vi "Parameter aktivieren.vi"(11 "Ref Anzeige":refnum<vi>[](array[refnum])) -> ()   [LabVIEW 2020, in "Anlagengrenzwerte.lvlib"]
uses:
  Anlagengrenzwerte.lvlib
  Passwortverwaltung/FGV Passwort Aktion.ctl
  Passwortverwaltung/Passwort.lvlib
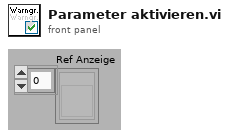
[diagram p1: front panel]
types:
  T1 = typedef "Passwort.lvlib/FGV Passwort Aktion.ctl" = enum16{"prüfen", "setzen", "Initialisieren", "PW speichern", "lesen", "PW Änderung"}
  T2 = cluster{cluster{"Soll aktiv":bool, "Warn Min aktiv":bool, "Warn Max aktiv":bool, "Abschalt Min aktiv":bool, "Abschalt Max aktiv":bool, "Regelung aktiv":bool}, cluster{"Soll aktiv":bool, "Warn Min aktiv":bool, "Warn Max aktiv":bool, "Abschalt Min aktiv":bool, "Abschalt Max aktiv":bool, "Regelung aktiv":bool}, cluster{"Soll aktiv":bool, "Warn Min aktiv":bool, "Warn Max aktiv":bool, "Abschalt Min aktiv":bool, "Abschalt Max aktiv":bool, "Regelung aktiv":bool}, cluster{"Soll aktiv":bool, "Warn Min aktiv":bool, "Warn Max aktiv":bool, "Abschalt Min aktiv":bool, "Abschalt Max aktiv":bool, "Regelung aktiv":bool}, cluster{"Soll aktiv":bool, "Warn Min aktiv":bool, "Warn Max aktiv":bool, "Abschalt Min aktiv":bool, "Abschalt Max aktiv":bool, "Regelung aktiv":bool}, cluster{"Soll aktiv":bool, "Warn Min aktiv":bool, "Warn Max aktiv":bool, "Abschalt Min aktiv":bool, "Abschalt Max aktiv":bool, "Regelung aktiv":bool}, cluster{"Soll aktiv":bool, "Warn Min aktiv":bool, "Warn Max aktiv":bool, "Abschalt Min aktiv":bool, "Abschalt Max aktiv":bool, "Regelung aktiv":bool}, cluster{"Soll aktiv":bool, "Warn Min aktiv":bool, "Warn Max aktiv":bool, "Abschalt Min aktiv":bool, "Abschalt Max aktiv":bool, "Regelung aktiv":bool}, cluster{"Soll aktiv":bool, "Warn Min aktiv":bool, "Warn Max aktiv":bool, "Abschalt Min aktiv":bool, "Abschalt Max aktiv":bool, "Regelung aktiv":bool}, cluster{"Soll aktiv":bool, "Warn Min aktiv":bool, "Warn Max aktiv":bool, "Abschalt Min aktiv":bool, "Abschalt Max aktiv":bool, "Regelung aktiv":bool}, cluster{"Soll aktiv":bool, "Warn Min aktiv":bool, "Warn Max aktiv":bool, "Abschalt Min aktiv":bool, "Abschalt Max aktiv":bool, "Regelung aktiv":bool}, cluster{"Soll aktiv":bool, "Warn Min aktiv":bool, "Warn Max aktiv":bool, "Abschalt Min aktiv":bool, "Abschalt Max aktiv":bool, "Regelung aktiv":bool}, cluster{"Soll aktiv":bool, "Warn Min aktiv":bool, "Warn Max aktiv":bool, "Abschalt Min aktiv":bool, "Abschalt Max aktiv":bool, "Regelung aktiv":bool}, cluster{"Soll aktiv":bool, "Warn Min aktiv":bool, "Warn Max aktiv":bool, "Abschalt Min aktiv":bool, "Abschalt Max aktiv":bool, "Regelung aktiv":bool}}
  T3 = cluster{"Soll aktiv":bool, "Warn Min aktiv":bool, "Warn Max aktiv":bool, "Abschalt Min aktiv":bool, "Abschalt Max aktiv":bool, "Regelung aktiv":bool}[]
  T4 = enum8{"Enabled", "Disabled", "Disabled and Grayed Out"}
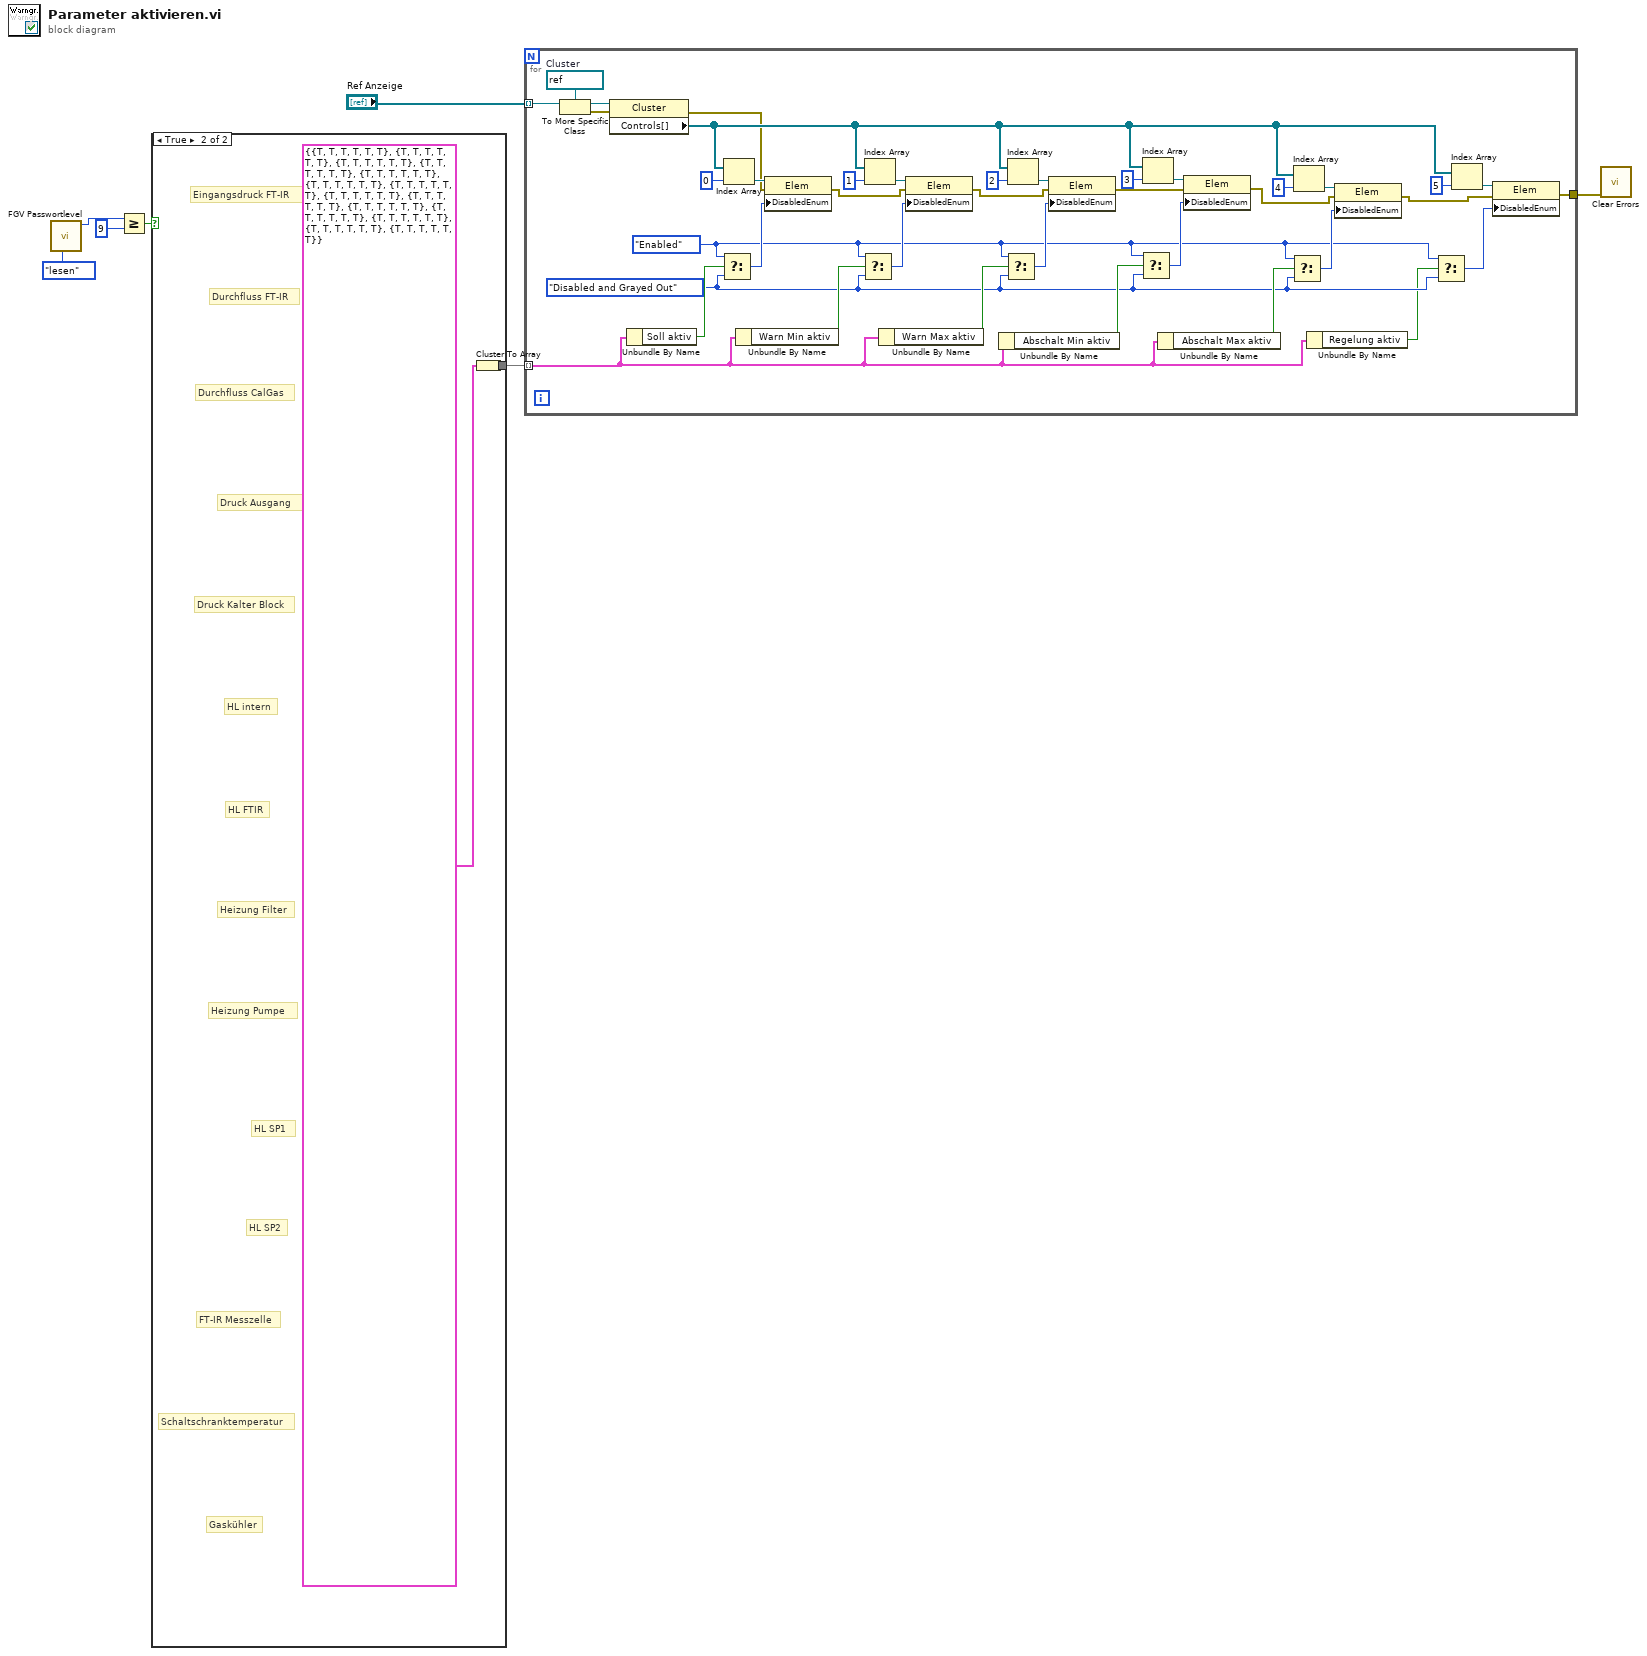
[diagram p0: block diagram]
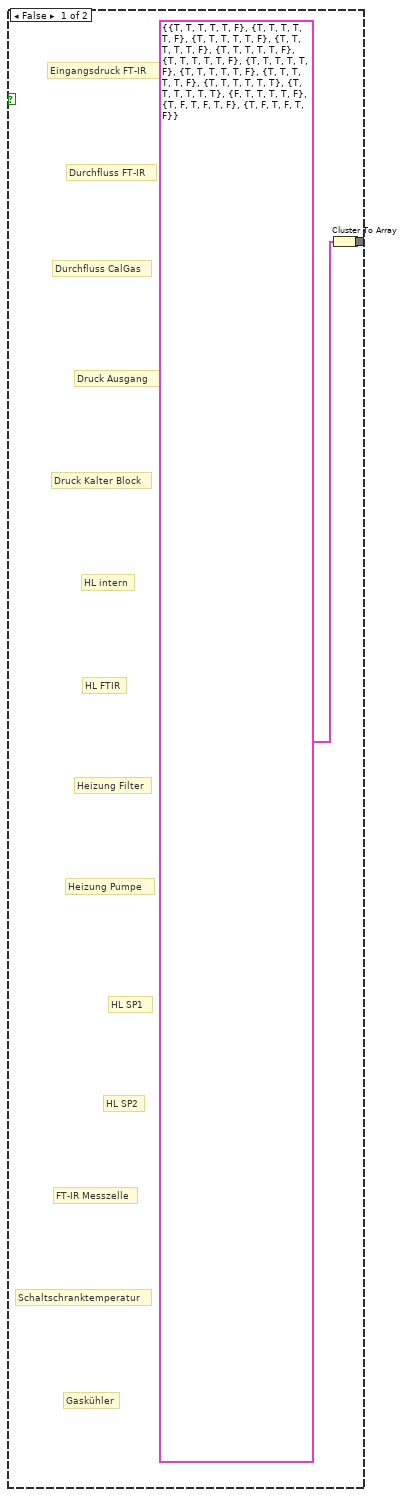
[diagram p2: hidden frame]
diagram:
  n1 = call "FGV Passwortlevel.vi"("FGV Passwort Aktion"=FGV_Passwort_Aktion."lesen") -> ("aktueller Level"=w3:i16)  [unwired: 8 in, 2 out]
  n2 = Greater Or Equal?(x=w3, y=i16 9) -> (x >= y?=w1:bool)
  n3 = case shown="True" w1 {
    tunnel: [w9 w11] -> w7
    frame False {
      # "HL FTIR"
      # "Durchfluss CalGas"
      # "Heizung Pumpe"
      # "Gaskühler"
      # "HL SP2"
      # "HL SP1"
      # "Schaltschranktemperatur"
      # "FT-IR Messzelle"
      # "Druck Ausgang"
      # "Heizung Filter"
      # "HL intern"
      # "Druck Kalter Block"
      # "Durchfluss FT-IR"
      # "Eingangsdruck FT-IR"
      n4 = Cluster To Array(cluster=T2 {{"Soll aktiv"=TRUE, "Warn Min aktiv"=TRUE, "Warn Max aktiv"=TRUE, "Abschalt Min aktiv"=TRUE, "Abschalt Max aktiv"=TRUE, "Regelung aktiv"=FALSE}, {"Soll aktiv"=TRUE, "Warn Min aktiv"=TRUE, "Warn Max aktiv"=TRUE, "Abschalt Min aktiv"=TRUE, "Abschalt Max aktiv"=TRUE, "Regelung aktiv"=FALSE}, {"Soll aktiv"=TRUE, "Warn Min aktiv"=TRUE, "Warn Max aktiv"=TRUE, "Abschalt Min aktiv"=TRUE, "Abschalt Max aktiv"=TRUE, "Regelung aktiv"=FALSE}, {"Soll aktiv"=TRUE, "Warn Min aktiv"=TRUE, "Warn Max aktiv"=TRUE, "Abschalt Min aktiv"=TRUE, "Abschalt Max aktiv"=TRUE, "Regelung aktiv"=FALSE}, {"Soll aktiv"=TRUE, "Warn Min aktiv"=TRUE, "Warn Max aktiv"=TRUE, "Abschalt Min aktiv"=TRUE, "Abschalt Max aktiv"=TRUE, "Regelung aktiv"=FALSE}, {"Soll aktiv"=TRUE, "Warn Min aktiv"=TRUE, "Warn Max aktiv"=TRUE, "Abschalt Min aktiv"=TRUE, "Abschalt Max aktiv"=TRUE, "Regelung aktiv"=FALSE}, {"Soll aktiv"=TRUE, "Warn Min aktiv"=TRUE, "Warn Max aktiv"=TRUE, "Abschalt Min aktiv"=TRUE, "Abschalt Max aktiv"=TRUE, "Regelung aktiv"=FALSE}, {"Soll aktiv"=TRUE, "Warn Min aktiv"=TRUE, "Warn Max aktiv"=TRUE, "Abschalt Min aktiv"=TRUE, "Abschalt Max aktiv"=TRUE, "Regelung aktiv"=FALSE}, {"Soll aktiv"=TRUE, "Warn Min aktiv"=TRUE, "Warn Max aktiv"=TRUE, "Abschalt Min aktiv"=TRUE, "Abschalt Max aktiv"=TRUE, "Regelung aktiv"=FALSE}, {"Soll aktiv"=TRUE, "Warn Min aktiv"=TRUE, "Warn Max aktiv"=TRUE, "Abschalt Min aktiv"=TRUE, "Abschalt Max aktiv"=TRUE, "Regelung aktiv"=TRUE}, {"Soll aktiv"=TRUE, "Warn Min aktiv"=TRUE, "Warn Max aktiv"=TRUE, "Abschalt Min aktiv"=TRUE, "Abschalt Max aktiv"=TRUE, "Regelung aktiv"=TRUE}, {"Soll aktiv"=FALSE, "Warn Min aktiv"=TRUE, "Warn Max aktiv"=TRUE, "Abschalt Min aktiv"=TRUE, "Abschalt Max aktiv"=TRUE, "Regelung aktiv"=FALSE}, {"Soll aktiv"=TRUE, "Warn Min aktiv"=FALSE, "Warn Max aktiv"=TRUE, "Abschalt Min aktiv"=FALSE, "Abschalt Max aktiv"=TRUE, "Regelung aktiv"=FALSE}, {"Soll aktiv"=TRUE, "Warn Min aktiv"=FALSE, "Warn Max aktiv"=TRUE, "Abschalt Min aktiv"=FALSE, "Abschalt Max aktiv"=TRUE, "Regelung aktiv"=FALSE}}) -> (array=w9:T3)
    }
    frame True {
      # "HL FTIR"
      # "Durchfluss CalGas"
      # "Heizung Pumpe"
      # "Gaskühler"
      # "HL SP2"
      # "HL SP1"
      # "Schaltschranktemperatur"
      # "FT-IR Messzelle"
      # "Druck Ausgang"
      # "Heizung Filter"
      # "HL intern"
      # "Druck Kalter Block"
      # "Durchfluss FT-IR"
      # "Eingangsdruck FT-IR"
      n5 = Cluster To Array(cluster=T2 {{"Soll aktiv"=TRUE, "Warn Min aktiv"=TRUE, "Warn Max aktiv"=TRUE, "Abschalt Min aktiv"=TRUE, "Abschalt Max aktiv"=TRUE, "Regelung aktiv"=TRUE}, {"Soll aktiv"=TRUE, "Warn Min aktiv"=TRUE, "Warn Max aktiv"=TRUE, "Abschalt Min aktiv"=TRUE, "Abschalt Max aktiv"=TRUE, "Regelung aktiv"=TRUE}, {"Soll aktiv"=TRUE, "Warn Min aktiv"=TRUE, "Warn Max aktiv"=TRUE, "Abschalt Min aktiv"=TRUE, "Abschalt Max aktiv"=TRUE, "Regelung aktiv"=TRUE}, {"Soll aktiv"=TRUE, "Warn Min aktiv"=TRUE, "Warn Max aktiv"=TRUE, "Abschalt Min aktiv"=TRUE, "Abschalt Max aktiv"=TRUE, "Regelung aktiv"=TRUE}, {"Soll aktiv"=TRUE, "Warn Min aktiv"=TRUE, "Warn Max aktiv"=TRUE, "Abschalt Min aktiv"=TRUE, "Abschalt Max aktiv"=TRUE, "Regelung aktiv"=TRUE}, {"Soll aktiv"=TRUE, "Warn Min aktiv"=TRUE, "Warn Max aktiv"=TRUE, "Abschalt Min aktiv"=TRUE, "Abschalt Max aktiv"=TRUE, "Regelung aktiv"=TRUE}, {"Soll aktiv"=TRUE, "Warn Min aktiv"=TRUE, "Warn Max aktiv"=TRUE, "Abschalt Min aktiv"=TRUE, "Abschalt Max aktiv"=TRUE, "Regelung aktiv"=TRUE}, {"Soll aktiv"=TRUE, "Warn Min aktiv"=TRUE, "Warn Max aktiv"=TRUE, "Abschalt Min aktiv"=TRUE, "Abschalt Max aktiv"=TRUE, "Regelung aktiv"=TRUE}, {"Soll aktiv"=TRUE, "Warn Min aktiv"=TRUE, "Warn Max aktiv"=TRUE, "Abschalt Min aktiv"=TRUE, "Abschalt Max aktiv"=TRUE, "Regelung aktiv"=TRUE}, {"Soll aktiv"=TRUE, "Warn Min aktiv"=TRUE, "Warn Max aktiv"=TRUE, "Abschalt Min aktiv"=TRUE, "Abschalt Max aktiv"=TRUE, "Regelung aktiv"=TRUE}, {"Soll aktiv"=TRUE, "Warn Min aktiv"=TRUE, "Warn Max aktiv"=TRUE, "Abschalt Min aktiv"=TRUE, "Abschalt Max aktiv"=TRUE, "Regelung aktiv"=TRUE}, {"Soll aktiv"=TRUE, "Warn Min aktiv"=TRUE, "Warn Max aktiv"=TRUE, "Abschalt Min aktiv"=TRUE, "Abschalt Max aktiv"=TRUE, "Regelung aktiv"=TRUE}, {"Soll aktiv"=TRUE, "Warn Min aktiv"=TRUE, "Warn Max aktiv"=TRUE, "Abschalt Min aktiv"=TRUE, "Abschalt Max aktiv"=TRUE, "Regelung aktiv"=TRUE}, {"Soll aktiv"=TRUE, "Warn Min aktiv"=TRUE, "Warn Max aktiv"=TRUE, "Abschalt Min aktiv"=TRUE, "Abschalt Max aktiv"=TRUE, "Regelung aktiv"=TRUE}}) -> (array=w11:T3)
    }
  }
  n6 = for {
    tunnel: "Ref Anzeige" -> [w48] mode=indexing
    tunnel: w7 -> [w23] mode=indexing
    tunnel: [w12] -> w5
    w24 = T4."Disabled and Grayed Out" ("Deaktiviert")
    w25 = T4."Enabled" ("Deaktiviert")
    w49 = refnum<vi> refnum  # Cluster
    n7 = To More Specific Class(target class=w49, reference=w48) -> (specific class reference=w50:refnum<vi>, error out=w19:errorcluster)  [unwired: 1 in]
    n8 = property class="Cluster"(reference=w50, error in=w19) -> (error out=w18:errorcluster, "Controls[]"=w20:refnum<vi>[])  [unwired: 1 out]
    n9 = Unbundle By Name(w23) -> ("Soll aktiv"=w38:bool)
    n10 = Select(t=w25, s=w38, f=w24) -> (s? t:f=w45:T4)
    n11 = Index Array(array=w20, index=0 ("Index")) -> (element=w46:refnum<vi>)
    n12 = Unbundle By Name(w23) -> ("Warn Min aktiv"=w37:bool)
    n13 = property class="Elem"(reference=w46, error in=w18, "DisabledEnum"=w45) -> (error out=w17:errorcluster)  [unwired: 1 out]
    n14 = Select(t=w25, s=w37, f=w24) -> (s? t:f=w44:T4)
    n15 = Index Array(array=w20, index=1 ("Index")) -> (element=w43:refnum<vi>)
    n16 = Unbundle By Name(w23) -> ("Warn Max aktiv"=w36:bool)
    n17 = property class="Elem"(reference=w43, error in=w17, "DisabledEnum"=w44) -> (error out=w16:errorcluster)  [unwired: 1 out]
    n18 = Unbundle By Name(w23) -> ("Abschalt Min aktiv"=w31:bool)
    n19 = Select(t=w25, s=w36, f=w24) -> (s? t:f=w41:T4)
    n20 = Index Array(array=w20, index=2 ("Index")) -> (element=w42:refnum<vi>)
    n21 = property class="Elem"(reference=w42, error in=w16, "DisabledEnum"=w41) -> (error out=w15:errorcluster)  [unwired: 1 out]
    n22 = Select(t=w25, s=w31, f=w24) -> (s? t:f=w35:T4)
    n23 = Index Array(array=w20, index=3 ("Index")) -> (element=w34:refnum<vi>)
    n24 = Unbundle By Name(w23) -> ("Abschalt Max aktiv"=w30:bool)
    n25 = property class="Elem"(reference=w34, error in=w15, "DisabledEnum"=w35) -> (error out=w14:errorcluster)  [unwired: 1 out]
    n26 = Select(t=w25, s=w30, f=w24) -> (s? t:f=w32:T4)
    n27 = Index Array(array=w20, index=4 ("Index")) -> (element=w33:refnum<vi>)
    n28 = Unbundle By Name(w23) -> ("Regelung aktiv"=w22:bool)
    n29 = property class="Elem"(reference=w33, error in=w14, "DisabledEnum"=w32) -> (error out=w13:errorcluster)  [unwired: 1 out]
    n30 = Select(t=w25, s=w22, f=w24) -> (s? t:f=w21:T4)
    n31 = Index Array(array=w20, index=5 ("Index")) -> (element=w26:refnum<vi>)
    n32 = property class="Elem"(reference=w26, error in=w13, "DisabledEnum"=w21) -> (error out=w12:errorcluster)  [unwired: 1 out]
  }
  n33 = call <vilib>:"Clear Errors.vi"("error in (no error)"=w5) -> ()  [unwired: 5 in, 2 out]
